vi "Read Pre AIV Values.vi"(8 "error in":errorcluster, 9 "R Load":dbl, 11 "DAC HeatFlow AIV in":refnum<class "DAC HeatFlow AOV.lvclass">) -> (0 "error out":errorcluster, 3 "DAC HeatFlow AIV out":refnum<class "DAC HeatFlow AOV.lvclass">)   [LabVIEW 2019, in "DAC.lvlib" / "DAC HeatFlow AOV.lvclass"]
uses:
  DAC HeatFlow AOV.lvclass
  DAC HeatFlow AOV.lvclass/DAC HeatFlow AOV.ctl
  <vilib>/DAQmx/read.llb/DAQmx Read (Analog Wfm 1Chan NSamp).vi
  <vilib>/Analysis/baseanly.llb/Mean (DBL).vi
  <vilib>/DAQmx/miscellaneous.llb/DAQmx Fill In Error Info.vi
  <vilib>/Analysis/NI_AALBase.lvlib
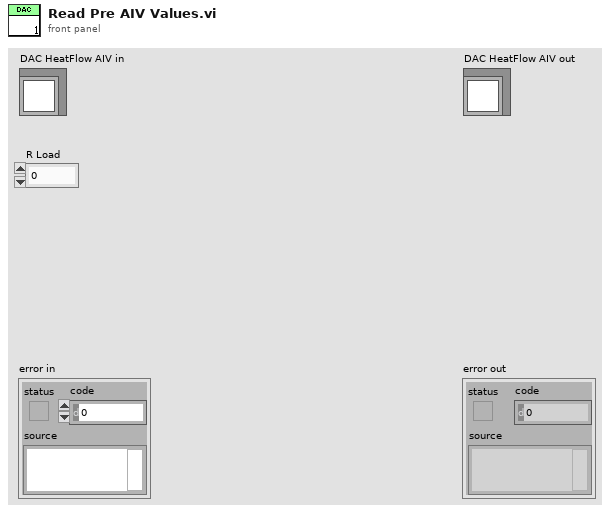
[diagram p1: front panel]
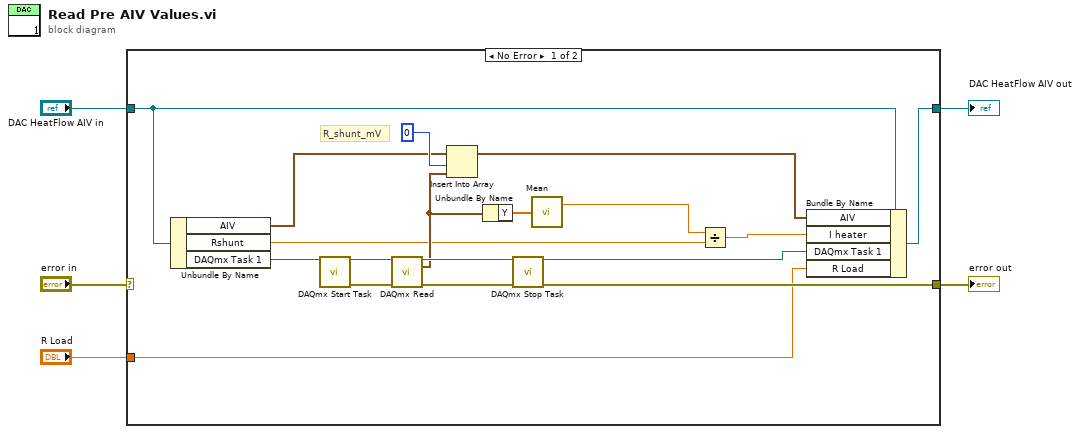
[diagram p0: block diagram]
diagram:
  n1 = case shown="No Error" "error in" {
    selector: "error in" -> [_ w25]
    tunnel: [w14 w25] -> w4
    tunnel: [w23 w24] -> w2
    tunnel: "DAC HeatFlow AIV in" -> [w22 w24]
    tunnel: "R Load" -> [w6 _]
    frame No Error {
      # "R_shunt_mV"
      n2 = Unbundle By Name(w22) -> ("AIV"=w8:waveform(dbl)[], "Rshunt"=w7:dbl, "DAQmx Task 1"=w21:refnum<k21>)
      n3 = call <vilib>:"DAQmx Start Task.vi"("task/channels in"=w21) -> ("task out"=w20:refnum<k21>, "error out"=w17:errorcluster)  [unwired: 13 in]
      n4 = call-poly <vilib>:"DAQmx Read.vi"("task/channels in"=w20, "error in"=w17) -> ("task out"=w19:refnum<k21>, "data"=w12:waveform(dbl), "error out"=w16:errorcluster)  [unwired: 11 in]
      n5 = Insert Into Array "Insert Into Array"(array=w8, index=0, new element=w12) -> (w13:waveform(dbl)[])
      n6 = Unbundle By Name(w12) -> ("Y"=w11:dbl[])
      n7 = call <vilib>:"DAQmx Stop Task.vi"("task/channels in"=w19, "error in"=w16) -> ("task out"=w18:refnum<k21>, "error out"=w14:errorcluster)  [unwired: 12 in]
      n8 = call-poly <vilib>:"Mean.vi"("X"=w11) -> ("mean"=w10:dbl)  [unwired: 1 out]
      n9 = Divide(x=w10, y=w7) -> (x/y=w9:dbl)
      n10 = Bundle By Name(cluster=w22, "AIV"=w13, "I heater"=w9, "DAQmx Task 1"=w18, "R Load"=w6) -> (w23:refnum<class "DAC HeatFlow AOV.lvclass">)
    }
    frame Error {
    }
  }
  "error out" <- w4
  "DAC HeatFlow AIV out" <- w2
